vi "X-CAN_Connection_Stream_Connection_EMG_Control.vi"() -> ()   [LabVIEW 2015]
uses:
  <vilib>/Stratom, Inc/X-CAN for myRIO (API)/X-CAN Class/Type Definitions/CAN_Speed.ctl
  <vilib>/Stratom, Inc/X-Modules for myRIO/Type Defs/MXPChannel.ctl
  <vilib>/Platform/TimedLoop/XDataNode/timing_clust.ctl
  <vilib>/Platform/TimedLoop/XDataNode/nitl_modes.ctl
  <vilib>/Platform/TimedLoop/XDataNode/wakeup.ctl
  <vilib>/platform/TimedLoop/XDataNode/XDataNode.xnode
  <vilib>/Stratom, Inc/X-CAN for myRIO (API)/X-CAN Class/X-CAN.lvclass
  <vilib>/Platform/TimedLoop/XDataNode/XDNodeRunTimeDep.lvlib
panel:
  out "Motor positions (degree)":T1(array[cluster]) {"Error Code (bits)" format="%b"}
  out "stop?":bool
  in  "Stop Button":bool
  # "REMEMBER: this subVI has always to be run as first."
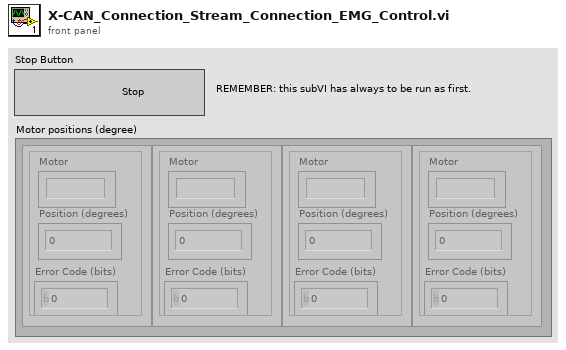
[diagram p1: front panel]
types:
  T1 = cluster{"Position (degrees)":i32, "Error Code (bits)":u8, "Motor":string}[]
  T2 = cluster{"Enable?":bool, "Reset?":bool, "EMG control":enum16{"Rest", "Biceps contracted", "Triceps contracted"}, "Motor speed":u8}
  T3 = typedef "MXPChannel.ctl" = enum16{"A/MXP", "B/MXP"}
  T4 = typedef "X-CAN.lvclass/CAN_Speed.ctl" = u8
  T5 = cluster{"ID":u8, "Position":u16, "Error Code":u8}[]
  T6 = typedef "XDNodeRunTimeDep.lvlib/timing_clust.ctl" = cluster{"Expected End [f-1]":u64, "Actual End [f-1]":u64, "Finished Late? [f-1]":bool, "Expected End [i-1]":u64, "Actual End [i-1]":u64, "Finished Late? [i-1]":bool, "Expected Start [i]":u64, "Actual Start [i]":u64, "Expected Start [f]":u64, "Actual Start [f]":u64, "Source Name":string, "Structure Name":string, "Period":i64, "Deadline":i64, "Offset":i64, "Start":i64, "Priority":i32, "Timeout":i32, "Mode":T7, "Wakeup Reason":T8, "Error":errorcluster, "Source Type":string, "Secondary Source Type":string, "Global End Time":u64, "Global Start Time":u64, "Frame Duration":u64, "Iteration Duration":u64, "Assigned CPU":i32, "I/O Scan Engine Mode":u32}
  T7 = typedef "XDNodeRunTimeDep.lvlib/nitl_modes.ctl" = enum32{"No Change", "Process missed periods, maintain original phase", "Discard missed periods, maintain original phase", "Process missed periods, ignore original phase", "Discard missed periods, ignore original phase"}
  T8 = typedef "XDNodeRunTimeDep.lvlib/wakeup.ctl" = enum32{"Normal", "Aborted", "Asynchronous wakeup", "Timing source error", "Timed loop error", "Timeout"}
  T9 = enum16{"Rest", "Biceps contracted", "Triceps contracted"}
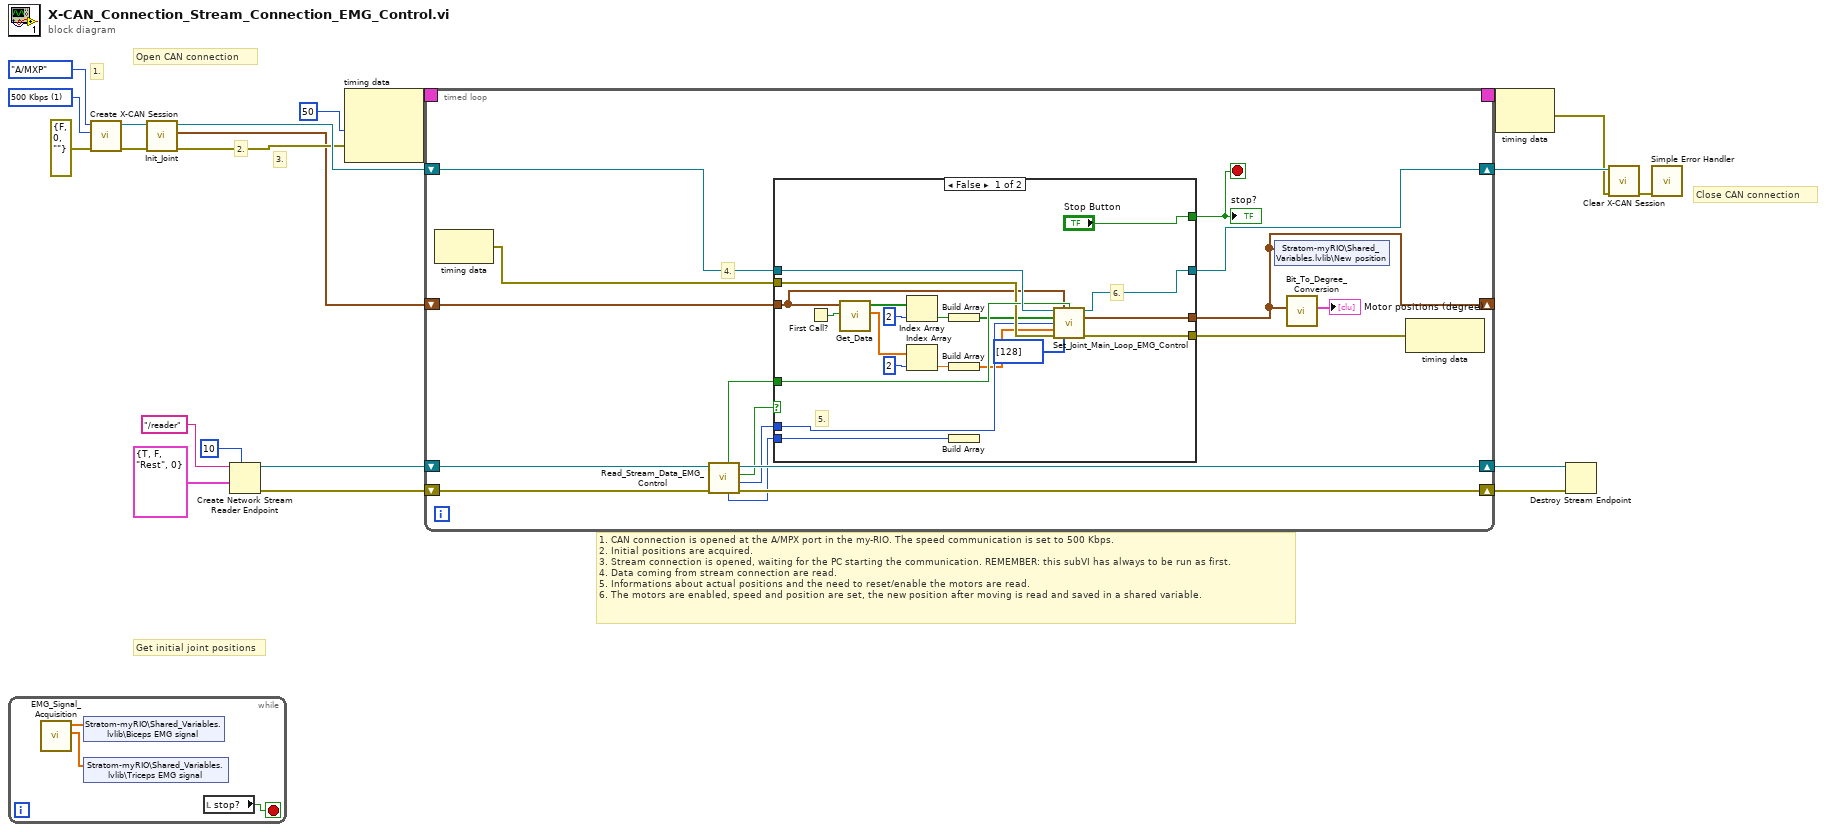
[diagram p0: block diagram]
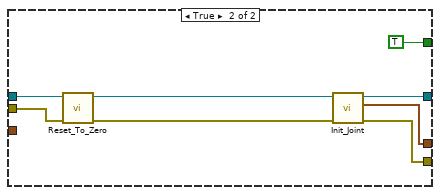
[diagram p2: hidden frame]
diagram:
  w20 = T4 1 items=["125 Kbps"=7, "250 Kbps"=3, "500 Kbps"=1, "1000 Kbps"=0, "95.238 Kbps"=6] ("CAN Speed [Kbps]")
  # "Close CAN connection"
  # "3."
  # "2."
  # "1."
  # "1. CAN connection is opened at the A/MPX port in the my-RIO. The speed communication is set to 500 Kbps.\n2. Initial positions are acquired.\n3. Stream connection is opened, waiting for the PC starting the communication. REMEMBER: this subVI has always to be run as first. \n4. Data coming from stream connection are read.\n5. Informations about actual positions and the need to reset/enable the motors are read.\n6. The motors are enabled, speed and position are set, the new position after moving is read and saved in a shared variable."
  # "Get initial joint positions"
  # "Open CAN connection"
  n1 = while {
    stop <- w24 stop-if-true
    n2 = call "EMG_Signal_Acquisition.vi"() -> ("Triceps EMG signal"=w22:dbl[], "Biceps EMG signal"=w23:dbl[])  [unwired: 10 in]
    n3 = shared-variable "Stratom-myRIO\\Shared_Variables.lvlib\\Biceps EMG signal"(w23) -> ()  [unwired: 1 in, 1 out]
    n4 = shared-variable "Stratom-myRIO\\Shared_Variables.lvlib\\Triceps EMG signal"(w22) -> ()  [unwired: 1 in, 1 out]
    n5 = local read "stop?"() -> (w24:bool)
  }
  n6 = call <vilib>:"Create X-CAN Session.vi"("error in (no error)"=errorcluster {"status"=FALSE, "code"=0, "source"=""}, "CAN Speed [Kbps]"=w20, "MXP Channel"=MXPChannel."A/MXP") -> ("error out"=w11:errorcluster, "X-CAN Session out"=w12:refnum<class "X-CAN.lvclass">)  [unwired: 7 in]
  n7 = call "Init_Joint.vi"("error in"=w11, "X-CAN Session in"=w12) -> ("error out"=w9:errorcluster, "Init Position"=w8:T5, "X-CAN Session out"=w10:refnum<class "X-CAN.lvclass">)  [unwired: 5 in, 1 out]
  n8 = Create Network Stream Reader Endpoint(7:10 ("reader buffer size"), 9:T2 {"Enable?"=TRUE, "Reset?"=FALSE, "EMG control"=enum."Rest", "Motor speed"=0} ("data in"), 11:"/reader" ("reader name")) -> (0:w2:errorcluster, 3:w3:refnum<k21>)  [unwired: 4 in]
  n9 = node-c288(i64 50 ("Period"), w9) -> (w18:T6)  [unwired: 1 in]
  n10 = timed-loop {
    timing: w18 -> [_]
    timing-out: [_] -> w17
    shift-right: [w37] -> w15
    shift-left: w10 -> [w40]
    shift-right: [w26] -> _
    shift-left: w8 -> [w36]
    shift-right: [w31] -> w6
    shift-left: w2 -> [w32]
    shift-right: [w33] -> w5
    shift-left: w3 -> [w34]
    stop <- w35 stop-if-true
    # "4."
    n11 = node-c288() -> (w39:errorcluster)  [unwired: 1 in]
    n12 = call "Read_Stream_Data_EMG_Control.vi"("error in (no error)"=w32, "endpoint in"=w34) -> ("error out"=w31:errorcluster, "EMG control"=w28:T9, "Reset to zero position?"=w30:bool, "endpoint out"=w33:refnum<k21>, "Motor speed (bit)"=w27:u8, "Enabled motor?"=w29:bool)  [unwired: 4 in]
    n13 = case shown="False" w30 {
      tunnel: w40 -> [w59 w68]
      tunnel: w39 -> [w57 w67]
      tunnel: [w56 w65] -> w38
      tunnel: [w53 w62] -> w37
      tunnel: [w54 w61] -> w26
      tunnel: w36 -> [w52 _]
      tunnel: ["Stop Button" TRUE ("stop")] -> w35
      tunnel: w29 -> [w58 _]
      tunnel: w28 -> [w51 _]
      tunnel: w27 -> [w42 _]
      frame False {
        # "6."
        # "5."
        n14 = First Call?() -> (First Call?: T/F=w55:bool)
        n15 = call "Get_Data.vi"("First Call?: T/F"=w55, "Init Position"=w52) -> ("Actual Positions"=w50:dbl[], "Reset Enable?"=w44:bool[])  [unwired: 8 in]
        n16 = Index Array(array=w44, index=2) -> (element=w45:bool)
        n17 = Index Array(array=w50, index=2) -> (element=w48:dbl)
        n18 = Build Array(w45) -> (w43:bool[])
        n19 = Build Array(w48) -> (w47:dbl[])
        n20 = Build Array(w42) -> ()  [unwired: 1 out]
        n21 = call "Set_Joint_Main_Loop_EMG_Control.vi"("X-CAN in"=w59, "Actual position"=w52, "Motor enabled?"=w58, "Reset?"=w43, "EMG control"=w51, "Current position"=w47, "error in (no error)"=w57, "Speed"=u16[] [128]) -> ("X-CAN out"=w53:refnum<class "X-CAN.lvclass">, "New position"=w54:T5, "error out"=w56:errorcluster)  [unwired: 5 in]
      }
      frame True {
        n22 = call "Reset_To_Zero.vi"("error in"=w67, "X-CAN Session in"=w68) -> ("error out"=w64:errorcluster, "X-CAN Session out"=w63:refnum<class "X-CAN.lvclass">)  [unwired: 8 in]
        n23 = call "Init_Joint.vi"("error in"=w64, "X-CAN Session in"=w63) -> ("error out"=w65:errorcluster, "Init Position"=w61:T5, "X-CAN Session out"=w62:refnum<class "X-CAN.lvclass">)  [unwired: 5 in, 1 out]
      }
    }
    "stop?" <- w35
    n24 = shared-variable "Stratom-myRIO\\Shared_Variables.lvlib\\New position"(w26) -> ()  [unwired: 1 in, 1 out]
    n25 = call "Bit_To_Degree_Conversion.vi"("Actual joints positions"=w26) -> ("Motor positions (degree)"=→"Motor positions (degree)":T1)  [unwired: 10 in]
    n26 = node-c288(w38) -> ()  [unwired: 1 out]
  }
  n27 = node-c288(w17) -> (w13:errorcluster)
  n28 = Destroy Stream Endpoint(8:w6, 11:w5) -> ()  [unwired: 1 out]
  n29 = call <vilib>:"Clear X-CAN Session.vi"("error in (no error)"=w13, "X-CAN Session in"=w15) -> ("error out"=w14:errorcluster)  [unwired: 9 in]
  n30 = call <vilib>:"Simple Error Handler.vi"("error in (no error)"=w14) -> ()  [unwired: 4 in, 5 out]
